vi "RPi WebDAV.vi"(8 "Error IN":errorcluster, 10 "RPi IP":string="10.31.176.22", 11 "Data Folder":path=path "c:/Closed_Data") -> (0 "Error OUT":errorcluster)   [LabVIEW 2013]
uses:
  <vilib>/WebDAVClient/Advanced/Put File.vi
  <vilib>/WebDAVClient/NI_WebDAV.lvlib
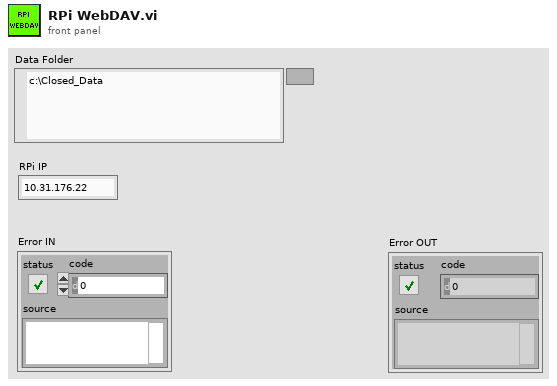
[diagram p1: front panel]
types:
  T1 = typedef "NI_WebDAV.lvlib/SessionHandle.ctl" = refnum<k1>
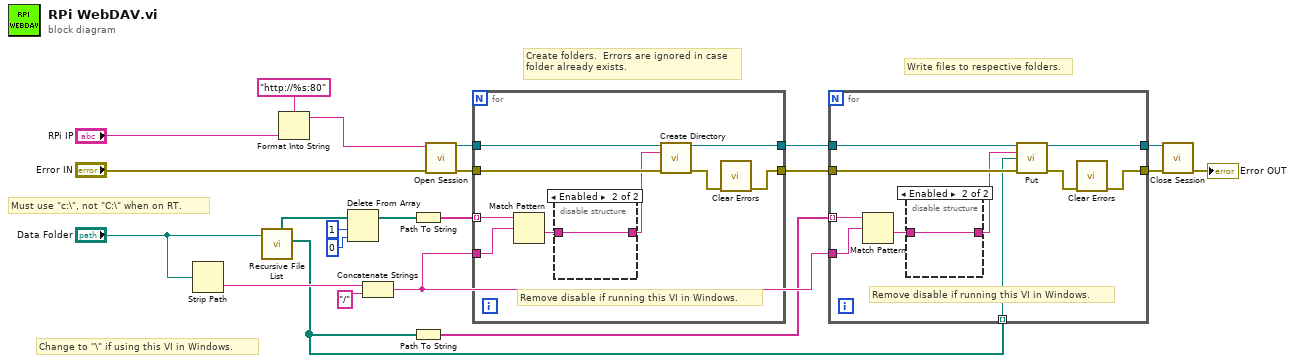
[diagram p0: block diagram]
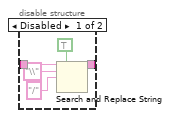
[diagram p2: hidden frame]
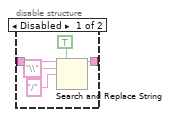
[diagram p3: hidden frame]
diagram:
  # "Change to \"\\\" if using this VI in Windows."
  # "Must use \"c:\\\", not \"C:\\\" when on RT."
  # "Write files to respective folders."
  # "Create folders.  Errors are ignored in case\nfolder already exists."
  n1 = Strip Path(path="Data Folder") -> (name=w17:string)  [unwired: 1 out]
  n2 = call <vilib>:"Recursive File List.vi"("Folder Path"="Data Folder") -> ("All Files in Dir"=w15:path[], "All Folders"=w22:path[])  [unwired: 6 in, 3 out]
  n3 = Format Into String(format string="http://%s:80" ("file uri"), "RPi IP") -> (resulting string=w10:string)  [unwired: 2 in, 1 out]
  n4 = Delete From Array(array=w22, length=1, index=0) -> (array with subset deleted=w19:path[])  [unwired: 1 out]
  n5 = Concatenate Strings(w17, "/" ("format string")) -> (w16:string)
  n6 = Path To String(path=w19) -> (string=w7:string[])
  n7 = Path To String(path=w15) -> (string=w4:string[])
  n8 = call <vilib>:"Open Session.vi"("host uri prefix"=w10, "error in (no error)"="Error IN") -> ("session handle out"=w8:T1, "error out"=w9:errorcluster)  [unwired: 12 in]
  n9 = for {
    tunnel: w9 -> [w30]
    tunnel: w8 -> [w29]
    tunnel: [w28] -> w6
    tunnel: [w27] -> w5
    tunnel: w7 -> [w26] mode=indexing
    tunnel: w16 -> [w25]
    # "Remove disable if running this VI in Windows."
    n10 = Match Pattern(string=w26, regular expression=w25) -> (after substring=w23:string)  [unwired: 1 in, 3 out]
    n11 = disable-structure shown="Enabled" {
      disable-tunnel: [w36 w37] -> w24
      disable-tunnel: w23 -> [w34 w37]
      frame Disabled {
        n12 = Search and Replace String(replace all?=TRUE ("replace all? (F)"), input string=w34, search string="\\", replace string="/" ("replace string (\"\")")) -> (result string=w36:string)  [unwired: 4 in, 3 out]
      }
      frame Enabled {
      }
    }
    n13 = call <vilib>:"Create Directory.vi"("session handle"=w29, "relative uri"=w24, "error in (no error)"=w30) -> ("session handle out"=w28:T1, "error out"=w31:errorcluster)  [unwired: 11 in]
    n14 = call <vilib>:"Clear Errors.vi"("error in (no error)"=w31) -> ("error out"=w27:errorcluster)  [unwired: 6 in]
  }
  n15 = for {
    tunnel: w5 -> [w46]
    tunnel: w6 -> [w45]
    tunnel: [w44] -> w3
    tunnel: [w43] -> w2
    tunnel: w4 -> [w42] mode=indexing
    tunnel: w16 -> [w41]
    tunnel: w15 -> [w39] mode=indexing
    # "Remove disable if running this VI in Windows."
    n16 = Match Pattern(string=w42, regular expression=w41) -> (after substring=w38:string)  [unwired: 1 in, 3 out]
    n17 = disable-structure shown="Enabled" {
      disable-tunnel: [w52 w53] -> w40
      disable-tunnel: w38 -> [w50 w53]
      frame Disabled {
        n18 = Search and Replace String(replace all?=TRUE ("replace all? (F)"), input string=w50, search string="\\", replace string="/" ("replace string (\"\")")) -> (result string=w52:string)  [unwired: 4 in, 3 out]
      }
      frame Enabled {
      }
    }
    n19 = call-poly <vilib>:"Put.vi"("session handle"=w45, "relative uri"=w40, "local file path"=w39, "error in (no error)"=w46) -> ("session handle out"=w44:T1, "error out"=w47:errorcluster)  [unwired: 9 in, 1 out]
    n20 = call <vilib>:"Clear Errors.vi"("error in (no error)"=w47) -> ("error out"=w43:errorcluster)  [unwired: 6 in]
  }
  n21 = call <vilib>:"Close Session.vi"("session handle"=w3, "error in (no error)"=w2) -> ("error out"=→"Error OUT":errorcluster)  [unwired: 13 in]
